vi "探头手动清洗.vi"(7 "校准参数":u16(ring) caption="校准参数：" items=["pH", "DO", "浊度", "电导率", "叶绿素a", "藻密度", "ORP", "DO2"], 8 "error in (no error)":errorcluster caption="错误输入（无错误）") -> (0 "error out":errorcluster caption="错误输出")   [LabVIEW 2016, in "斯坦道多参数.lvlib"]
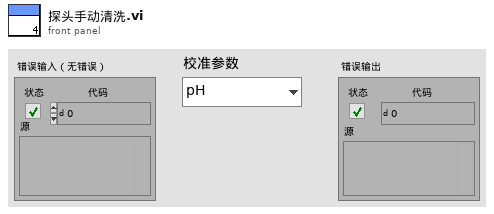
[diagram p1: front panel]
types:
  T1 = typedef "斯坦道多参数.lvlib/探头类型.ctl" = enum16{"禹山", "国弘", "纳清", "STD"}
  T2 = enum16{"NULL", "pH", "Cond", "DO", "Turb", "ORP"}
  T3 = enum16{"NULL", "pH", "Cond", "DO", "Turb", "ORP", "6", "7", "8", "9", "氯化物"}
  T4 = enum16{"null", "pH", "DO", "浊度", "电导率", "叶绿素a", "藻密度"}
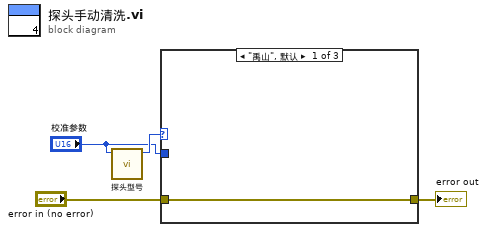
[diagram p0: block diagram]
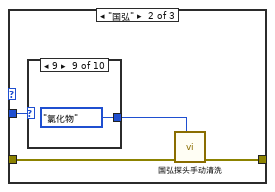
[diagram p2: hidden frame]
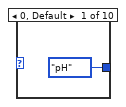
[diagram p3: hidden frame]
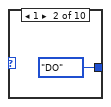
[diagram p4: hidden frame]
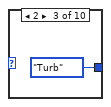
[diagram p5: hidden frame]
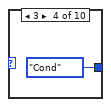
[diagram p6: hidden frame]
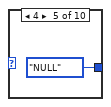
[diagram p7: hidden frame]
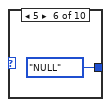
[diagram p8: hidden frame]
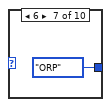
[diagram p9: hidden frame]
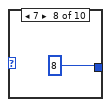
[diagram p10: hidden frame]
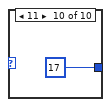
[diagram p11: hidden frame]
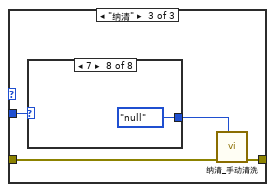
[diagram p12: hidden frame]
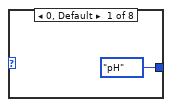
[diagram p13: hidden frame]
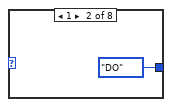
[diagram p14: hidden frame]
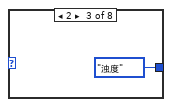
[diagram p15: hidden frame]
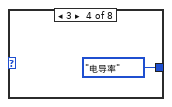
[diagram p16: hidden frame]
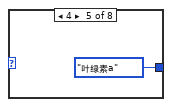
[diagram p17: hidden frame]
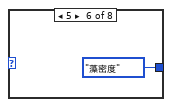
[diagram p18: hidden frame]
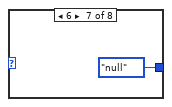
[diagram p19: hidden frame]
diagram:
  n1 = call "探头型号.vi"("校准参数"="校准参数") -> ("探头型号"=w4:T1)  [unwired: 8 in, 2 out]
  n2 = case shown="\"禹山\", 默认" w4 {
    tunnel: "校准参数" -> [_ w9 w23]
    tunnel: "error in (no error)" -> [w5 w8 w21]
    tunnel: [w5 w6 w20] -> w1
    frame "禹山", Default {
    }
    frame "国弘" {
      n3 = case shown="9" w9 {
        tunnel: [T2."pH" ("探头") T2."DO" ("探头") T2."Turb" ("探头") T2."Cond" ("探头") T2."NULL" ("探头") T2."NULL" ("探头") T2."ORP" ("探头") 8 T3."氯化物" ("探头") 17 ("探头")] -> w7
        frame 0, Default {
        }
        frame 1 {
        }
        frame 2 {
        }
        frame 3 {
        }
        frame 4 {
        }
        frame 5 {
        }
        frame 6 {
        }
        frame 7 {
        }
        frame 9 {
        }
        frame 11 {
        }
      }
      n4 = call "国弘探头手动清洗.vi"("探头"=w7, "error in (no error)"=w8) -> ("error out"=w6:errorcluster)  [unwired: 8 in, 1 out]
    }
    frame "纳清" {
      n5 = case shown="7" w23 {
        tunnel: [T4."pH" ("探头") T4."DO" ("探头") T4."浊度" ("探头") T4."电导率" ("探头") T4."叶绿素a" ("探头") T4."藻密度" ("探头") T4."null" ("探头") T4."null" ("探头")] -> w22
        frame 0, Default {
        }
        frame 1 {
        }
        frame 2 {
        }
        frame 3 {
        }
        frame 4 {
        }
        frame 5 {
        }
        frame 6 {
        }
        frame 7 {
        }
      }
      n6 = call "纳清_手动清洗.vi"("探头"=w22, "error in (no error)"=w21) -> ("error out"=w20:errorcluster)  [unwired: 9 in]
    }
  }
  "error out" <- w1
